vi "HardWare Config Variables.vi"() -> (2 "HardWare_Phsical Channels Config.vi":T3)   [LabVIEW 2016]
uses:
  HardWare/Ctrls/HardWare _ Channel Configurations PopUp Type.ctl
  ToolKit/Popup/Private/Ctrls/POP_Data Type.ctl
panel:
  # "TreeDisCols：显示在tree控件上的\n参数第一列对应参数名，第二列为显示名称"
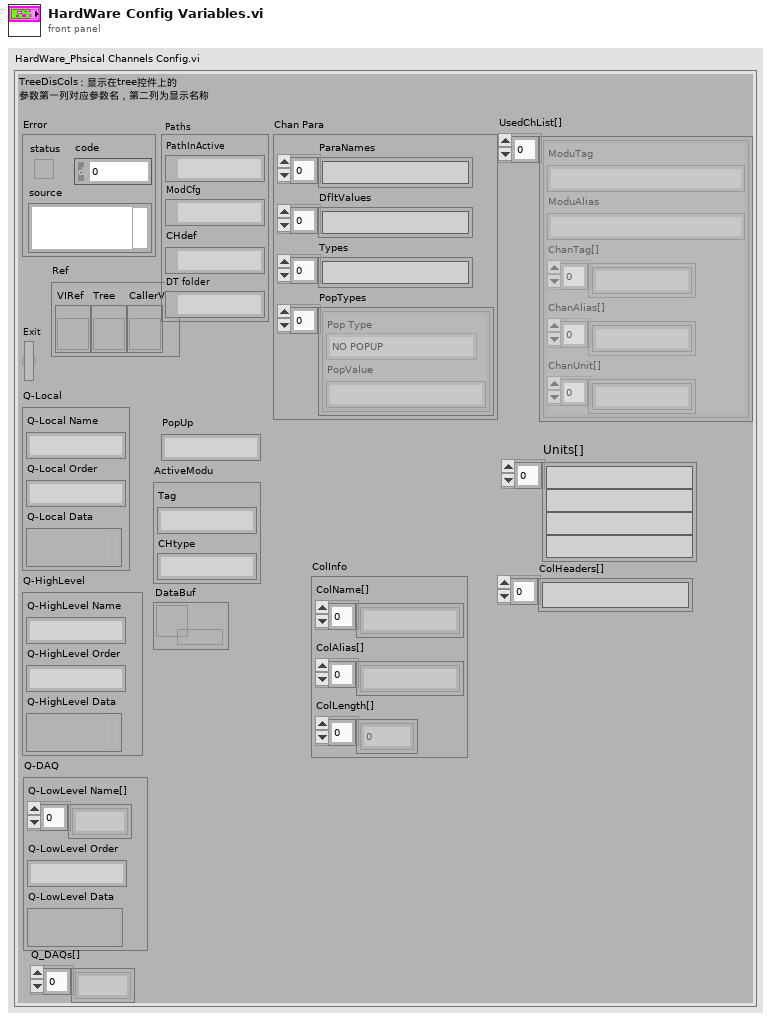
[diagram p1: front panel]
types:
  T1 = typedef "HardWare _ Channel Configurations PopUp Type.ctl" = cluster{"Pop Type":T2, "PopValue":string}
  T2 = typedef "POP_Data Type.ctl" = enum16{"NO POPUP", "Unkown", "String", "Integer", "Float", "Color", "Boolean", "Ring", "Captioned String", "Captioned Integer", "Button Color", "2 Int Cluster", "4 Int Cluster", "6-Dbl Cluster", "Path", "Combox", "Time", "ShotCut String"}
  T3 = cluster{"Error":errorcluster, "Ref":cluster{"VIRef":refnum<vi>, "Tree":refnum<vi>, "CallerVI":refnum<vi>}, "Exit":bool, " Paths":cluster{"PathInActive":path, "ModCfg":path, "CHdef":path, "DT folder":path}, "Q-Local":cluster{"Q-Local Name":string, "Q-Local Order":string, "Q-Local Data":variant}, "Q-HighLevel":cluster{"Q-HighLevel Name":string, "Q-HighLevel Order":string, "Q-HighLevel Data":variant}, "Q-DAQ":cluster{"Q-LowLevel Name[]":string[], "Q-LowLevel Order":string, "Q-LowLevel Data":variant}, "PopUp":string, "Chan Para":cluster{"ParaNames":string[], "DfltValues":string[], "Types":string[], "PopTypes":T1[]}, "Q_DAQs[]":string[], "ActiveModu":cluster{"Tag":string, "CHtype":string}, "ColInfo":cluster{"ColName[]":string[], "ColAlias[]":string[], "ColLength[]":i32[]}, "UsedChList[]":cluster{"ModuTag":string, "ModuAlias":string, "ChanTag[]":string[], "ChanAlias[]":string[], "ChanUnit[]":string[]}[], "DataBuf":refnum<queue>, "Units[]":string[], "ColHeaders[]":string[]}
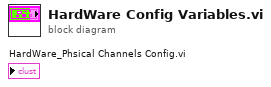
[diagram p0: block diagram]
diagram:
